vi "Configure Protection.vi"(6 "Protection (None)":T1, 8 "error in":errorcluster, 10 "Limit":dbl, 11 "4124 in":refnum<class "4124.lvclass">) -> (0 "error out":errorcluster, 3 "4124 out":refnum<class "4124.lvclass">)   [LabVIEW 2018, in "4124.lvlib" / "4124.lvclass"]
doc: "Configure Protection setting, available options:\n\n0: None\n1: Over Voltage\n2: Under Voltage\n3: Over Current\n\nDbl Precision Limit"
uses:
  4124.lvclass
  builds/Power_Supply.lvlibp/Custom Control/Protection.ctl
  <instrlib>/NI RMX-412x Power Supplies/NI RMX-412x Power Supplies.lvlib
  builds/Power_Supply.lvlibp/Power Supply.lvclass
  C:/Users/Ron.Dexter.LUMINARTECH/Desktop/builds/Power_Supply.lvlibp/Power Supply.lvclass
  builds/Power_Supply.lvlibp
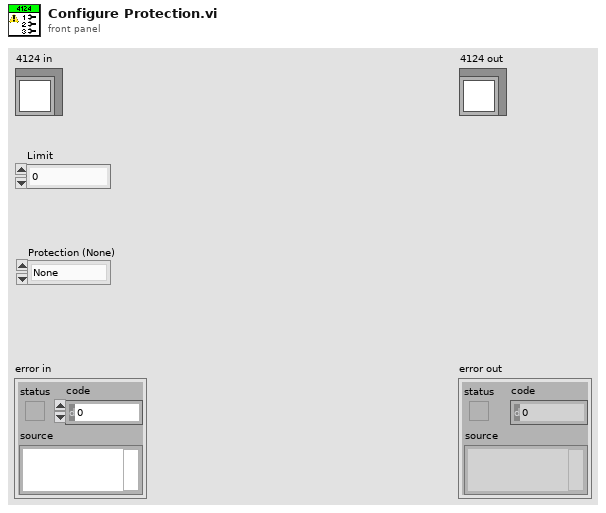
[diagram p1: front panel]
types:
  T1 = typedef "Power_Supply.lvlibp/Protection.ctl" = enum16{"None", "Over Volt", "Under Volt", "Over Current"}
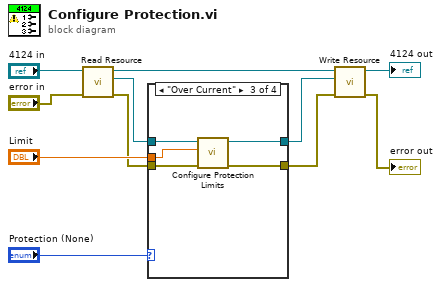
[diagram p0: block diagram]
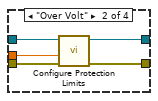
[diagram p3: hidden frame]
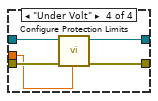
[diagram p4: hidden frame]
diagram:
  n1 = call "Read Resource.vi"("error in"="error in", "Power Supply in"="4124 in") -> ("error out"=w4:errorcluster, "Resource"=w2:refnum<visa-resource-name>, "Power Supply out"=w9:refnum<class "4124.lvclass">)  [unwired: 7 in]
  n2 = case shown="\"Over Current\"" "Protection (None)" {
    tunnel: "Limit" -> [_ w18 w19 w24]
    tunnel: w4 -> [w13 w17 w23 w28]
    tunnel: [w13 w16 w22 w27] -> w3
    tunnel: w2 -> [w12 w15 w21 w26]
    tunnel: [w12 w14 w20 w25] -> w1
    frame "None", Default {
    }
    frame "Over Volt" {
      n3 = call <instrlib>:"Configure Protection Limits.vi"("error in (no error)"=w17, "Overvoltage Protection Limit (0)"=w18, "VISA resource name"=w15) -> ("error out"=w16:errorcluster, "VISA resource name out"=w14:refnum<visa-resource-name>)  [unwired: 7 in]
    }
    frame "Over Current" {
      n4 = call <instrlib>:"Configure Protection Limits.vi"("error in (no error)"=w23, "Overcurrent Protection Limit (0)"=w19, "VISA resource name"=w21) -> ("error out"=w22:errorcluster, "VISA resource name out"=w20:refnum<visa-resource-name>)  [unwired: 7 in]
    }
    frame "Under Volt" {
      n5 = call <instrlib>:"Configure Protection Limits.vi"("Low Voltage Limit (0)"=w24, "error in (no error)"=w28, "VISA resource name"=w26) -> ("error out"=w27:errorcluster, "VISA resource name out"=w25:refnum<visa-resource-name>)  [unwired: 7 in]
    }
  }
  n6 = call "Write Resource.vi"("error in"=w3, "Resource"=w1, "Power Supply in"=w9) -> ("error out"=→"error out":errorcluster, "Power Supply out"=→"4124 out":refnum<class "4124.lvclass">)  [unwired: 7 in]
